vi "DO Post Step Type.vi"(8 "error in (no error)":errorcluster, 9 "DOWrite":T1, 10 "Socket No":u16=1, 11 "NI Digital Output in":refnum<class "NI Digital Output.lvclass">) -> (0 "error out":errorcluster, 2 "PhysicalChannel":string[](array[string]), 3 "NI Digital Output out":refnum<class "NI Digital Output.lvclass">)   [LabVIEW 2023, in "HardwareAbstractionLayer_LVOOP.lvlib" / "NI Digital Output.lvclass"]
uses:
  NI Digital Output.lvclass
  DO_class/DO DAQ/Control/DO Write Enable.ctl
  NI Digital Output.lvclass/NI Digital Output.ctl
  Database/Database.lvclass
  <resource>/objmgr/daqmx.rc
  DO_class/DO.lvclass
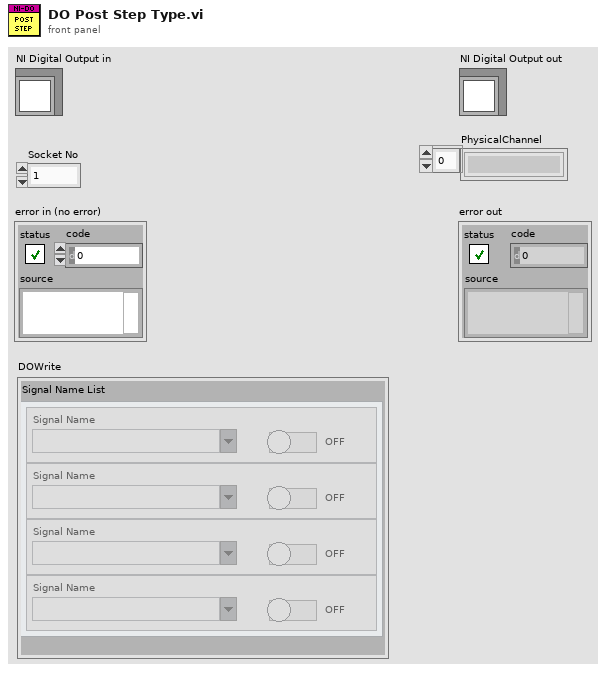
[diagram p1: front panel]
types:
  T1 = typedef "HardwareAbstractionLayer_LVOOP.lvlib/DO.lvclass/DO Write Enable.ctl" = cluster{"Signal Name List":cluster{"Signal Name":string, "Enable Output":bool}[]}
  T2 = cluster{"table":string, "condition":string, "columns":string[]}
  T3 = cluster{"Signal Name":string, "Enable Output":bool}[]
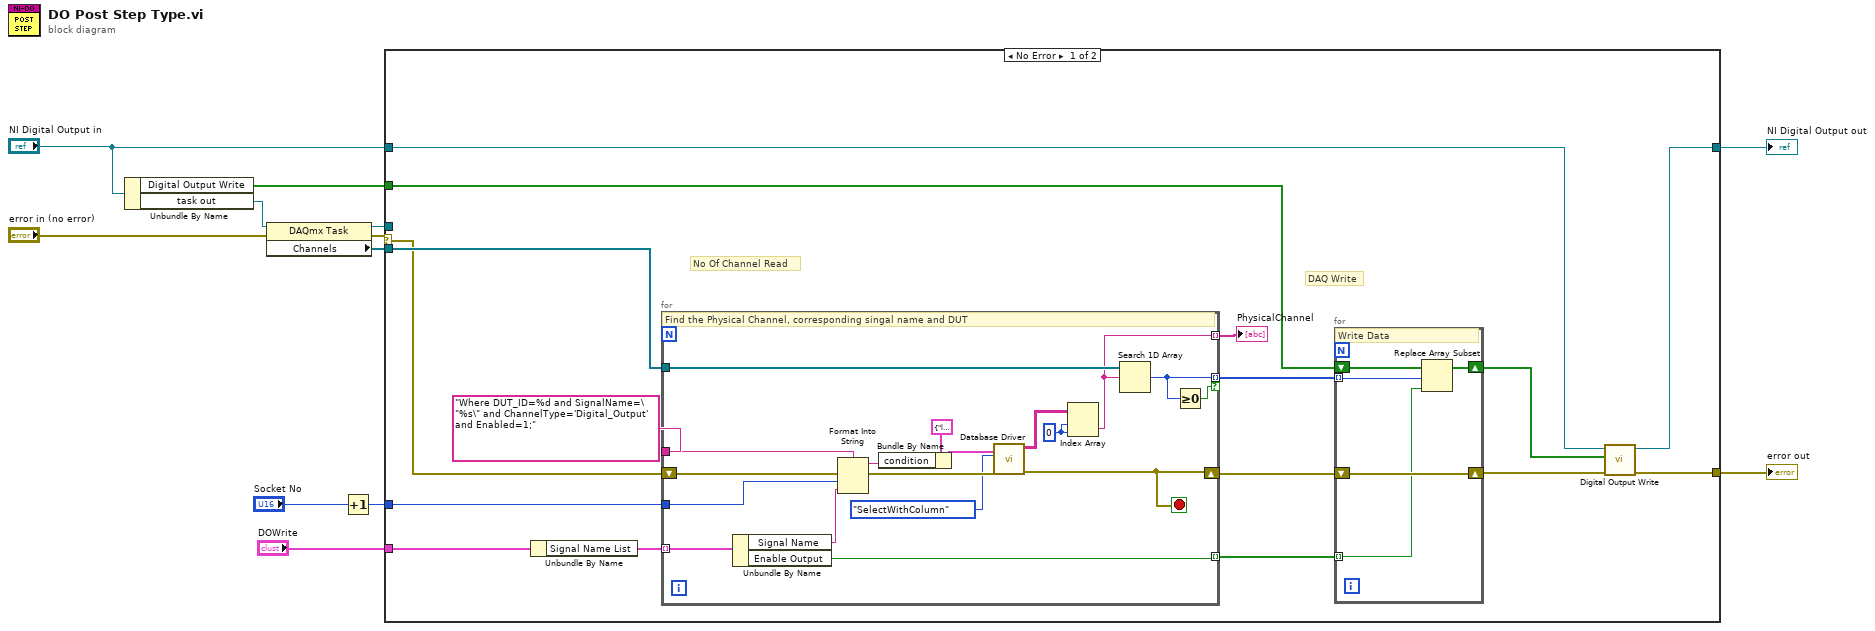
[diagram p0: block diagram]
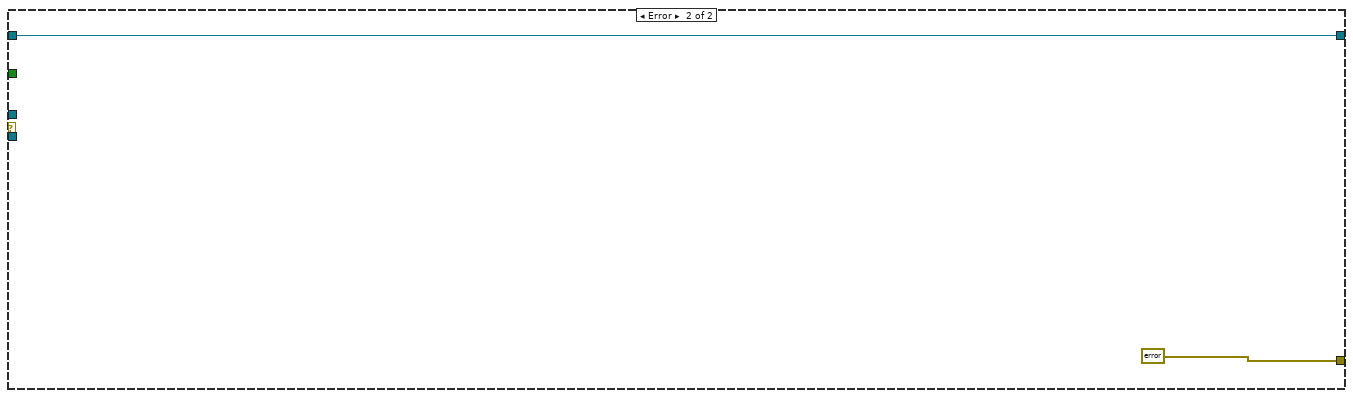
[diagram p2: hidden frame]
diagram:
  n1 = Unbundle By Name("NI Digital Output in") -> ("Digital Output Write"=w5:bool[], "task out"=w12:refnum<k21>)
  n2 = property class="DAQmx Task"(reference=w12, error in="error in (no error)") -> (reference out=w9:refnum<k21>, error out=w6:errorcluster, "Channels"=w8:refnum<k21>[])
  n3 = Increment(x="Socket No") -> (x+1=w10:u16)
  n4 = case shown="No Error" w6 {
    selector: w6 -> [w22 _]
    tunnel: [w16 errorcluster {"status"=TRUE, "code"=0, "source"="AO Task is not been created. please check in database."} ("error constant")] -> w2
    tunnel: w9 -> [_ _]
    tunnel: w8 -> [w24 _]
    tunnel: w10 -> [w23 _]
    tunnel: w5 -> [w20 _]
    tunnel: "NI Digital Output in" -> [w19 w52]
    tunnel: [w15 w52] -> w3
    tunnel: "DOWrite" -> [w14 _]
    frame No Error {
      # "No Of Channel Read"
      # "DAQ Write"
      n5 = Unbundle By Name(w14) -> ("Signal Name List"=w28:T3)
      n6 = for {
        tunnel: w28 -> [w32] mode=indexing
        tunnel: "Where DUT_ID=%d and SignalName=\"%s\" and ChannelType='Digital_Output' and Enabled=1;" -> [w46]
        shift-right: [w35] -> w21
        shift-left: w22 -> [w42]
        tunnel: w24 -> [w39]
        tunnel: [w37] -> w26 mode=indexing if=w36
        tunnel: w23 -> [w34]
        tunnel: [w30] -> w25 mode=indexing
        tunnel: [w29] -> w13 mode=indexing
        stop <- w35 stop-if-true
        w38 = 0 ("disabled index (col)")
        # "Find the Physical Channel, corresponding singal name and DUT"
        n7 = Unbundle By Name(w32) -> ("Signal Name"=w31:string, "Enable Output"=w30:bool)
        n8 = Format Into String(format string=w46, error in=w42, w34, w31) -> (resulting string=w44:string, error out=w41:errorcluster)  [unwired: 1 in]
        n9 = Bundle By Name(cluster=T2 {"table"="ltt.daq_configuration", "condition"="Where ChannelType='Analog_Input' and Enabled=1", "columns"=["PhysicalChannel"]} ("SQLTableData"), "condition"=w44) -> (w43:T2)
        n10 = call "Database Driver.vi"("SQLTableData"=w43, "error in"=w41, "Select"=enum16{"SelectWithQuery", "SelectWithColumn"}."SelectWithColumn") -> ("error out"=w35:errorcluster, "data"=w40:string[][])  [unwired: 5 in, 2 out]
        n11 = Index Array(array=w40, index (row)=w38, index (col)=w38) -> (element=w29:string)
        n12 = Search 1D Array(1D array=w39, element=w29) -> (index of element=w37:i32)  [unwired: 1 in]
        n13 = Greater Or Equal To 0?(x=w37) -> (x >= 0?=w36:bool)
      }
      "PhysicalChannel" <- w13
      n14 = for {
        shift-right: [w51] -> w18
        shift-left: w21 -> [w51]
        tunnel: w26 -> [w50] mode=indexing
        tunnel: w25 -> [w47] mode=indexing
        shift-right: [w48] -> w17
        shift-left: w20 -> [w49]
        # "Write Data"
        n15 = Replace Array Subset(array=w49, new element=w47, index=w50) -> (w48:bool[])
      }
      n16 = call-dynamic "Digital Output Write.vi"("error in"=w18, "Digital Output Write"=w17, "NI Digital Output in"=w19) -> ("error out"=w16:errorcluster, "NI Digital Output out"=w15:refnum<class "NI Digital Output.lvclass">)  [unwired: 7 in]
    }
    frame Error {
    }
  }
  "error out" <- w2
  "NI Digital Output out" <- w3
